vi "Car Position Actual Update.vi"(8 "error in (no error)":errorcluster, 10 "Car Position Actual":u8, 11 "Car Position Monitor Model in":refnum<class "Simulated Car Position Monitor Model.lvclass">) -> (0 "error out":errorcluster, 3 "Car Position Monitor Model out":refnum<class "Simulated Car Position Monitor Model.lvclass">)   [LabVIEW 2019, in "Simulated Car Position Monitor Model.lvclass"]
uses:
  <vilib>/gpm_packages/@cs/Car-wash/Source/Simulated Car Position Monitor Model/Simulated Car Position Monitor Model.lvclass
  <vilib>/gpm_packages/@cs/Car-wash/Source/Simulated Car Position Monitor Model/Simulated Car Position Monitor Model.lvclass/Simulated Car Position Monitor Model.ctl
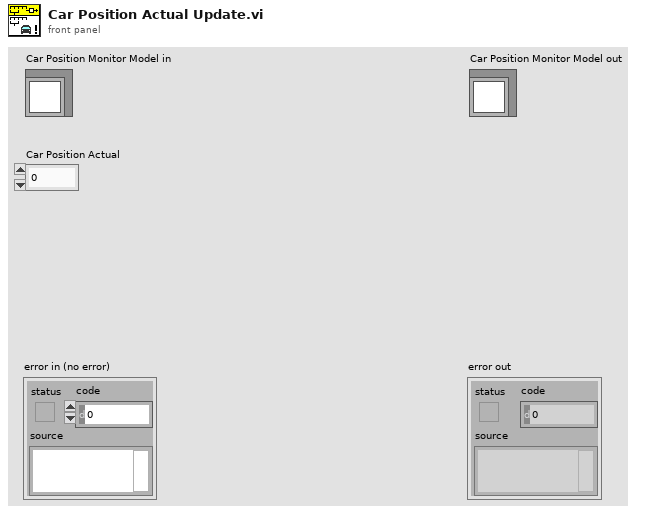
[diagram p1: front panel]
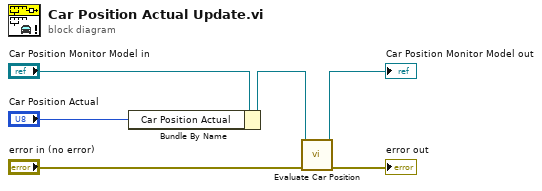
[diagram p0: block diagram]
diagram:
  n1 = Bundle By Name(cluster="Car Position Monitor Model in", "Car Position Actual"="Car Position Actual") -> (w4:refnum<class "Simulated Car Position Monitor Model.lvclass">)
  n2 = call <vilib>:"Evaluate Car Position.vi"("error in (no error)"="error in (no error)", "Car Position Monitor Model in"=w4) -> ("error out"=→"error out":errorcluster, "Car Position Monitor Model out"=→"Car Position Monitor Model out":refnum<class "Simulated Car Position Monitor Model.lvclass">)  [unwired: 8 in]
